vi "Emballage_BDD_GPAO_V_ARTICLE_FILTRE.vi"(0 "NOVALVE_FILTRE":string, 1 "tbl_ID_ARTICLE":string[](array[string]), 5 "indice_produit":string, 7 "Melange_des_lots_possible":string, 9 "Affiche_code_barre":string, 11 "error in (no error)":errorcluster, 12 "Famille":string) -> (4 "Donnée Final":string[][](array[string]), 6 "Colonne":string[](array[string])=["NOS_ARTICLE", "SUFFIXE", "CLC_DESIGNATION", "INDICE_REV", "ENR_ANNULE", "NB_PIECE_EMB", "REVIS_SUFF"], 8 "Donnée":string[][](array[string]), 15 "error out":errorcluster)   [LabVIEW 2020]
uses:
  Modules/FS/60_FS_Controles/60_FS_SetGet.ctl
  <vilib>/addons/database/Connection.llb/DB Tools Open Connec (Path).vi
  <vilib>/addons/database/Connection.llb/Conn Execute.vi
  <vilib>/addons/database/Recordset.llb/Rec Fetch Recordset Data (R).vi
  <vilib>/addons/database/Recordset.llb/Rec Destroy - Connection.vi
  <vilib>/addons/database/NI_Database_API.lvlib
panel:
  out "sep_code_barre_indice":string
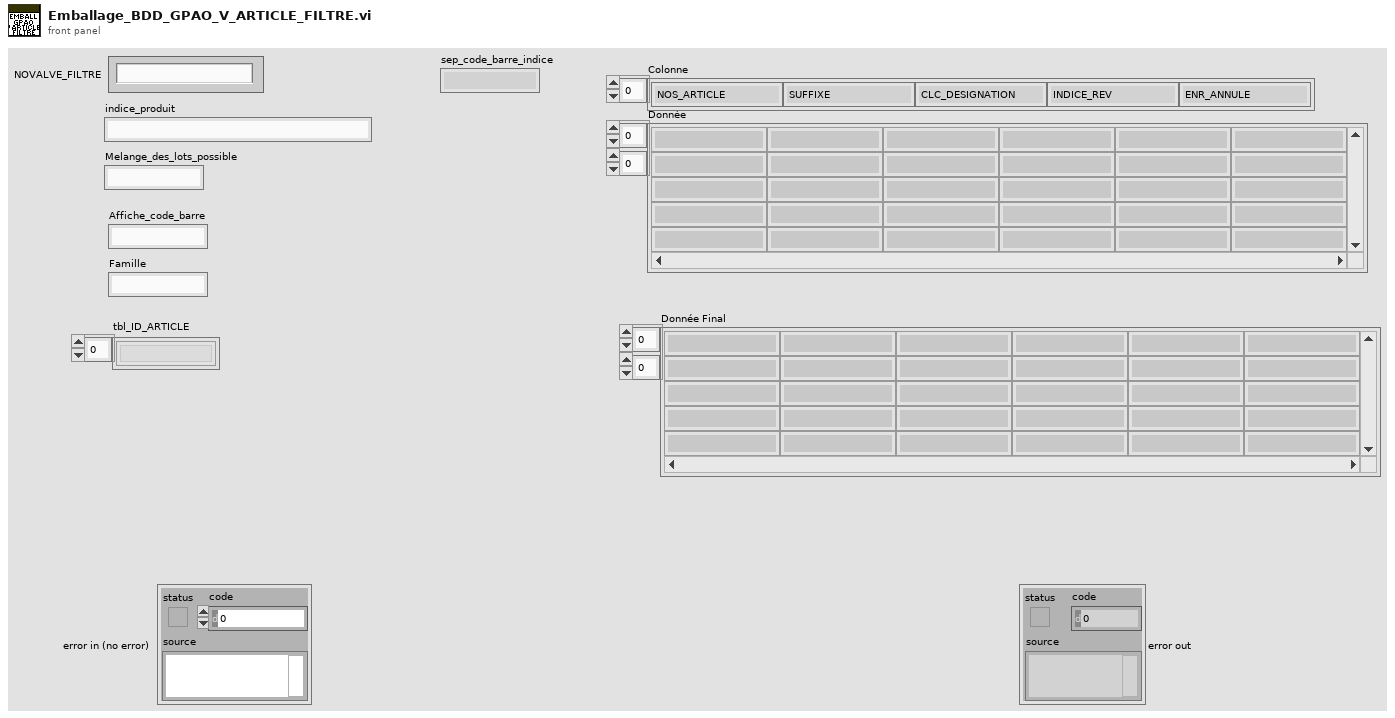
[diagram p1: front panel]
types:
  T1 = typedef "60_FS_SetGet.ctl" = enum16{"set", "get"}
  T2 = typedef "60_FS_CLT_Chemins.ctl" = cluster{"Racine_local":path, "Racine_reseau":path, "Racine_Support_Application":path, "Fichier_Journalisation":path, "Connexion_BDD_VSX":path, "Connexion_BDD_PLZ":path}
  T3 = typedef "NI_Database_API.lvlib/Conn ObjectReference.ctl" = refnum<k1>
  T4 = typedef "NI_Database_API.lvlib/Rec ObjectReference.ctl" = refnum<k1>
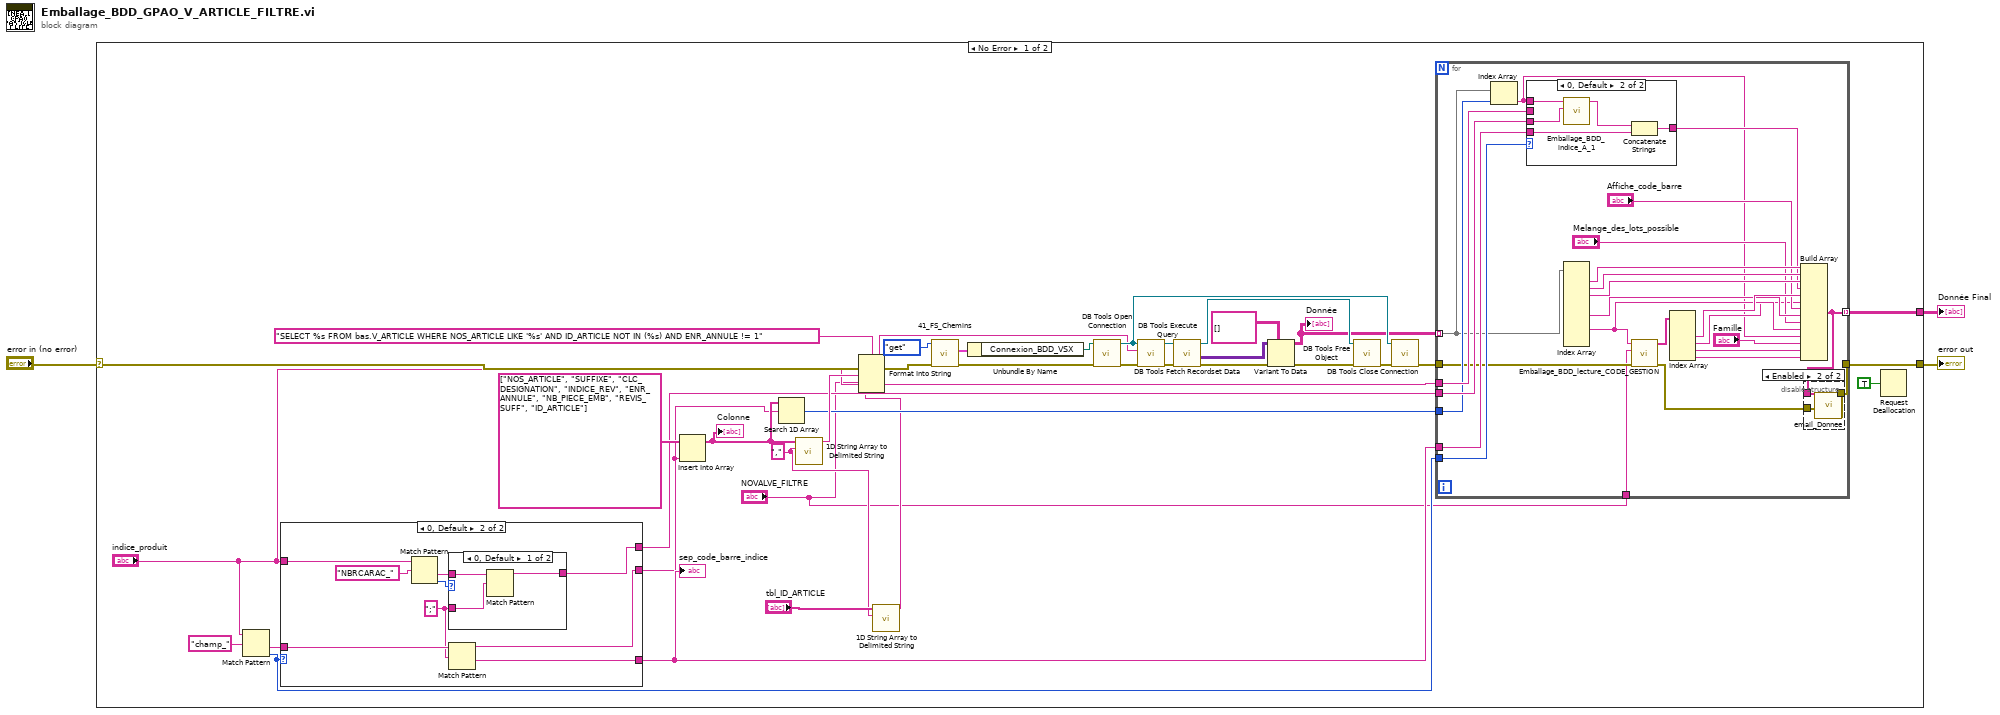
[diagram p0: block diagram]
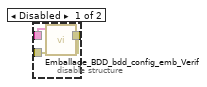
[diagram p2: hidden frame]
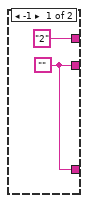
[diagram p4: hidden frame]
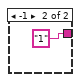
[diagram p5: hidden frame]
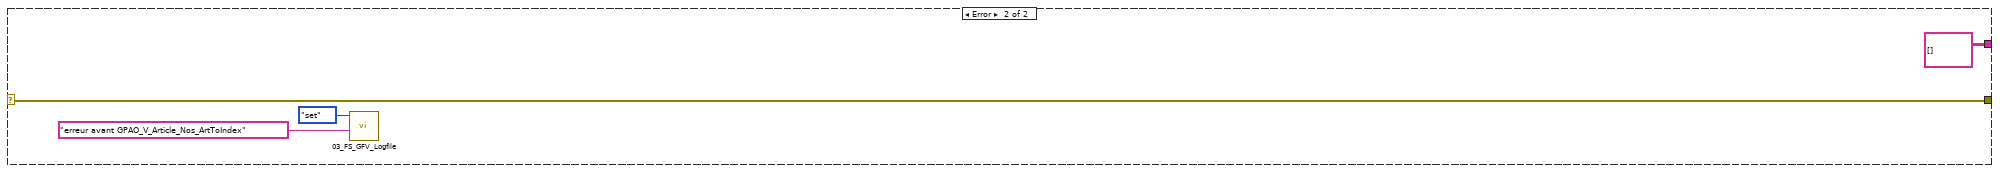
[diagram p6: hidden frame]
diagram:
  n1 = case shown="No Error" "error in (no error)" {
    selector: "error in (no error)" -> [w26 w98]
    tunnel: [w9 w98] -> w2
    tunnel: [w12 string[][] [] ("Chaînes []")] -> w1
    frame No Error {
      w7 = "," ("delimiter")
      n2 = Match Pattern(string="indice_produit", regular expression="champ_" ("expression régulière")) -> (after substring=w23:string, offset past match=w16:i32)  [unwired: 1 in, 2 out]
      n3 = case shown="0, Default" w16 {
        tunnel: w23 -> [_ w90]
        tunnel: [w81 w89] -> w21
        tunnel: [w81 w88] -> w19
        tunnel: "indice_produit" -> [_ w87]
        tunnel: ["2" ("indice_produit") w83] -> w18
        frame -1 {
          w81 = ""
        }
        frame 0, Default {
          w84 = ";" ("expression régulière")
          n4 = Match Pattern(string=w87, regular expression="NBRCARAC_" ("expression régulière")) -> (after substring=w85:string, offset past match=w82:i32)  [unwired: 1 in, 2 out]
          n5 = case shown="0, Default" w82 {
            tunnel: w85 -> [w93 _]
            tunnel: w84 -> [w92 _]
            tunnel: [w91 "1" ("indice_produit")] -> w83
            frame 0, Default {
              n6 = Match Pattern(string=w93, regular expression=w92) -> (before substring=w91:string)  [unwired: 1 in, 3 out]
            }
            frame -1 {
            }
          }
          n7 = Match Pattern(string=w90, regular expression=w84) -> (before substring=w88:string, after substring=w89:string)  [unwired: 1 in, 2 out]
        }
      }
      "sep_code_barre_indice" <- w21
      n8 = Insert Into Array(array=string[] ["NOS_ARTICLE", "SUFFIXE", "CLC_DESIGNATION", "INDICE_REV", "ENR_ANNULE", "NB_PIECE_EMB", "REVIS_SUFF", "ID_ARTICLE"], new element=w19) -> (w20:string[])  [unwired: 1 in]
      "Colonne" <- w20
      n9 = Search 1D Array(1D array=w20, element=w19) -> (index of element=w17:i32)  [unwired: 1 in]
      n10 = call <vilib>:"1D String Array to Delimited String.vi"("delimiter"=w7, "string array"=w20) -> ("delimited string"=w27:string)  [unwired: 9 in]
      n11 = call <vilib>:"1D String Array to Delimited String.vi"("delimiter"=w7, "string array"="tbl_ID_ARTICLE") -> ("delimited string"=w5:string)  [unwired: 9 in]
      n12 = Format Into String(format string="SELECT %s FROM bas.V_ARTICLE WHERE NOS_ARTICLE LIKE '%s' AND ID_ARTICLE NOT IN (%s) AND ENR_ANNULE != 1" ("Requète"), error in=w26, w27, "NOVALVE_FILTRE", w5) -> (resulting string=w28:string, error out=w25:errorcluster)  [unwired: 1 in]
      n13 = call "41_FS_Chemins.vi"("error in (no error)"=w25, "SetGet"=60_FS_SetGet."get") -> ("error out"=w39:errorcluster, "CLT_Chemins_out"=w40:T2)  [unwired: 8 in]
      n14 = Unbundle By Name(w40) -> ("Connexion_BDD_VSX"=w33:path)
      n15 = call-poly <vilib>:"DB Tools Open Connection.vi"("error in (no error)"=w39, "connection information"=w33) -> ("error out"=w31:errorcluster, "connection reference"=w32:T3)  [unwired: 6 in]
      n16 = call-poly <vilib>:"DB Tools Execute Query.vi"("error in (no error)"=w31, "SQL query"=w28, "connection reference"=w32) -> ("error out"=w38:errorcluster, "recordset reference"=w37:T4)  [unwired: 5 in]
      n17 = call-poly <vilib>:"DB Tools Fetch Recordset Data.vi"("error in (no error)"=w38, "recordset reference"=w37) -> ("error out"=w34:errorcluster, "recordset data"=w35:variant[][], "recordset reference out"=w14:T4)  [unwired: 3 in]
      n18 = Variant To Data(error in=w34, type=string[][] [] ("Chaînes []"), Variant=w35) -> (data=w11:string[][], error out=w15:errorcluster)
      "Donnée" <- w11
      n19 = call-poly <vilib>:"DB Tools Free Object.vi"("error in (no error)"=w15, "recordset reference"=w14) -> ("error out"=w13:errorcluster)  [unwired: 8 in, 1 out]
      n20 = call <vilib>:"DB Tools Close Connection.vi"("error in (no error)"=w13, "connection reference"=w32) -> ("error out"=w10:errorcluster)  [unwired: 5 in]
      n21 = for {
        tunnel: w11 -> [w62] mode=indexing
        tunnel: w21 -> [w67]
        tunnel: w18 -> [w66]
        tunnel: "indice_produit" -> [w65]
        tunnel: w17 -> [w63]
        tunnel: w16 -> [w64]
        tunnel: [w44] -> w12 mode=indexing
        tunnel: w10 -> [w61]
        tunnel: [w42] -> w9
        tunnel: "NOVALVE_FILTRE" -> [w45]
        n22 = Index Array(array=w62, index=w63) -> (element=w46:string)
        n23 = case shown="0, Default" w64 {
          tunnel: w65 -> [w74 _]
          tunnel: [w74 w77] -> w47
          tunnel: w46 -> [_ w79]
          tunnel: w67 -> [_ w76]
          tunnel: w66 -> [_ w75]
          frame -1 {
          }
          frame 0, Default {
            n24 = call "Emballage_BDD_indice_A_1.vi"("NbrDeCar."=w75, "indiceLettre"=w79) -> ("indiceAttenduNum"=w78:string)  [unwired: 9 in]
            n25 = Concatenate Strings(w78, w76) -> (w77:string)
          }
        }
        n26 = Index Array(array=w62) -> (element #1=w59:string, element #2=w58:string, element #3=w57:string, element #6=w54:string, element #8=w52:string)  [unwired: 10 in, 5 out]
        n27 = call "Emballage_BDD_lecture_CODE_GESTION.vi"("Error in"=w61, "NOVALVE_FILTRE"=w45, "ID_ARTICLE_GPAO"=w52) -> ("Error out"=w43:errorcluster, "données"=w60:string[])  [unwired: 7 in]
        n28 = Index Array(array=w60) -> (element #2=w56:string, element #3=w48:string, element #4=w50:string, element #5=w49:string)  [unwired: 5 in, 1 out]
        n29 = Build Array(w59, w58, w57, w47, w56, w48, "Affiche_code_barre", w54, "Melange_des_lots_possible", w52, w46, "Famille", w50, w49) -> (w44:string[])
        n30 = disable-structure shown="Enabled" {
          disable-tunnel: w44 -> [w70 w71]
          disable-tunnel: w43 -> [w69 w73]
          disable-tunnel: [w68 w72] -> w42
          frame Disabled {
            n31 = call "Emballage_BDD_bdd_config_emb_Verif.vi"("Error in"=w69, "tableau_config"=w70) -> ("Error out"=w68:errorcluster)  [unwired: 9 in]
          }
          frame Enabled {
            n32 = call "email_Donnee.vi"("entrée d'erreur (pas d'erreur)"=w73, "tableau_config"=w71) -> ("sortie d'erreur"=w72:errorcluster)  [unwired: 9 in]
          }
        }
      }
      n33 = Request Deallocation(TRUE ("flag")) -> ()
    }
    frame Error {
      n34 = call "03_FS_GFV_Logfile.vi"("Chaîne"="erreur avant GPAO_V_Article_Nos_ArtToIndex", "States"=60_FS_SetGet."set") -> ()  [unwired: 8 in, 2 out]
    }
  }
  "error out" <- w2
  "Donnée Final" <- w1
